vi "Load SCM Waveform Data.vi"(4 "error in":errorcluster, 5 "# Records":i32, 6 "# Records to Skip":i32, 7 "Source File":path) -> (0 "error out":errorcluster, 3 "Data":waveform(dbl)[][](array[waveform]))   [LabVIEW 2012]
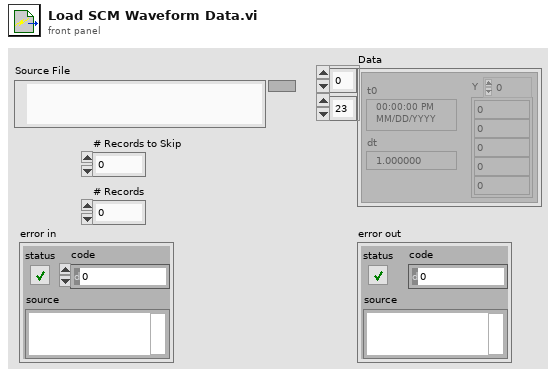
[diagram p1: front panel]
types:
  T1 = enum16{"big-endian, network order", "native, host order", "little-endian"}
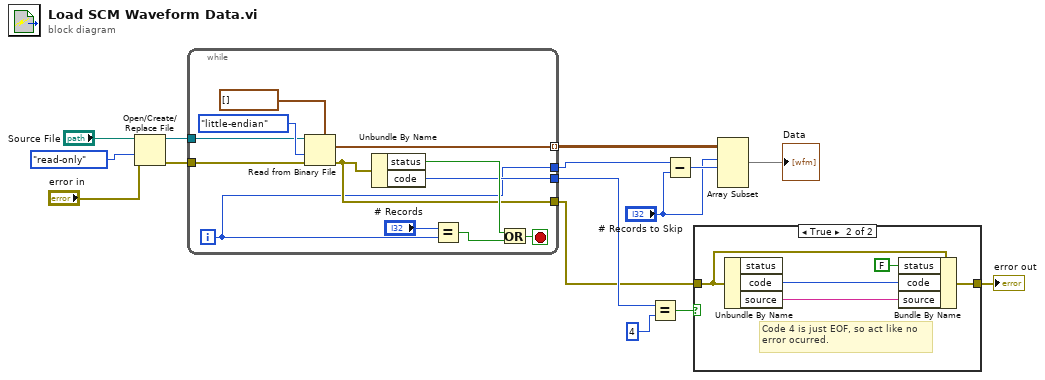
[diagram p0: block diagram]
diagram:
  n1 = Open/Create/Replace File(file path (use dialog)="Source File", error in="error in", access (0:read/write)=enum16{"read/write", "read-only", "write-only"}."read-only") -> (refnum out=w12:refnum<file>, error out=w11:errorcluster)  [unwired: 3 in, 1 out]
  n2 = while {
    tunnel: [w22] -> w10 mode=indexing
    tunnel: [w23] -> w6
    tunnel: w12 -> [w19]
    tunnel: w11 -> [w18]
    tunnel: [w17] -> w5
    tunnel: [w16] -> w2
    i -> [w16]
    stop <- w26 stop-if-true
    n3 = Read from Binary File(5:waveform(dbl)[] [] ("Difference"), 8:w18, 9:T1."little-endian" ("byte order (0:big-endian, network order)"), 11:w19) -> (0:w17:errorcluster, 2:w22:waveform(dbl)[])  [unwired: 2 in, 2 out]
    n4 = Unbundle By Name(w17) -> ("status"=w25:bool, "code"=w23:i32)
    n5 = Equal?(x="# Records", y=w16) -> (x = y?=w24:bool)
    n6 = Or(x=w25, y=w24) -> (x .or. y?=w26:bool)
  }
  n7 = Equal?(x=w6, y=4 ("code")) -> (x = y?=w8:bool)
  n8 = Subtract(x=w2, y="# Records to Skip") -> (x-y=w3:i32)
  n9 = case shown="True" w8 {
    tunnel: w5 -> [w28 w33]
    tunnel: [w28 w29] -> w4
    frame False {
    }
    frame True {
      # "Code 4 is just EOF, so act like no\nerror ocurred."
      n10 = Unbundle By Name(w33) -> ("code"=w32:i32, "source"=w31:string)  [unwired: 1 out]
      n11 = Bundle By Name(cluster=w33, "status"=FALSE, "code"=w32, "source"=w31) -> (w29:errorcluster)
    }
  }
  "error out" <- w4
  n12 = Array Subset(array=w10, index (row)="# Records to Skip", length (row)=w3) -> (→"Data":waveform(dbl)[][])  [unwired: 2 in]
